vi "Periodic Tasks.vi"(8 "error in (no error)":errorcluster) -> ()   [LabVIEW 2016]
doc: "This VI runs in parallel to other tasks. It can contain as many user-defined periodic loops as you need. These can carry out PID or other sorts of timed response."
uses:
  <vilib>/Rock Robotics/WPI/Utilities/WPI_GetSetVariantRefNum.vi
panel:
  in  "Far Away (2)":u32(colorbox)=16775840
  in  "Far Away":u32(colorbox)=65282
  in  "Lower Value":u32(colorbox)=65282
  in  "Within Limit Distance":u32(colorbox)=65282
  in  "Limit Distance from Sensor":u8(slide)=80 scale=0.0..100.0
  out "sensor":dbl
  out "output variable":dbl
  out "Voltage":dbl
  in  "LED_Off":u32(colorbox)=16775840
  in  "Position Speed":u32(slide)=20 scale=5.0..2000.0
  in  "LED_On":u32(colorbox)=65282
  in  "LED Position":u8(slide)=7 scale=0.0..30.0
  in  "Brightness":u8(slide)=255 scale=0.0..255.0
  out "error out":errorcluster
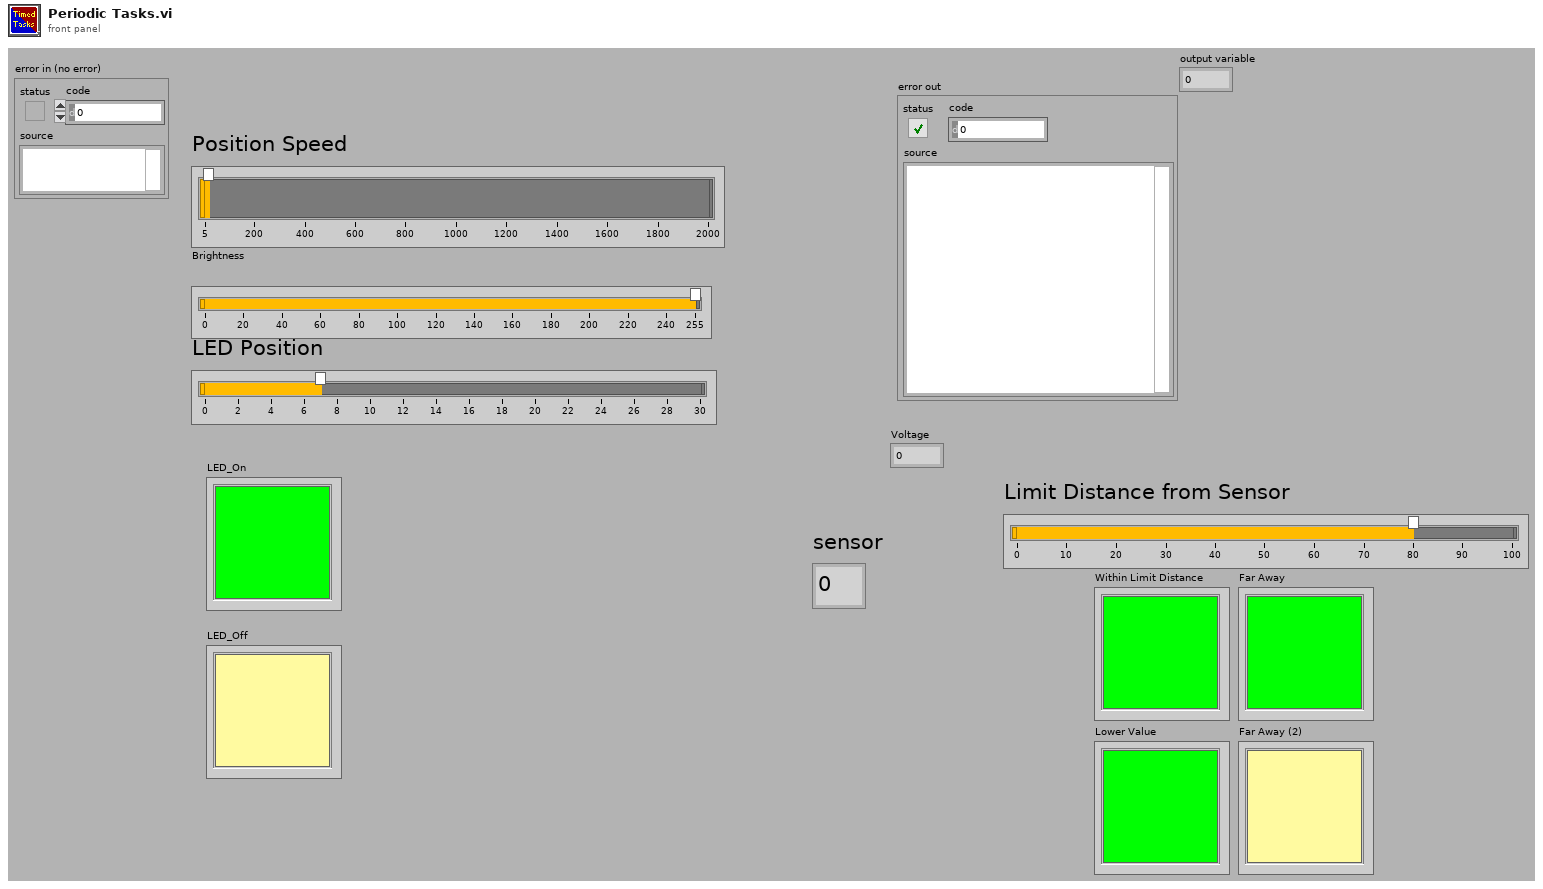
[diagram p1: front panel]
types:
  T1 = typedef "WPI_JoystickDevRef.ctl" = cluster{"Device":T2}
  T2 = typedef "WPI_JoystickDeviceEnum.ctl" = enum16{"USB 0", "USB 1", "USB 2", "USB 3", "USB 4", "USB 5"}
  T3 = typedef "WPI_RobotDriveDevRef.ctl" = cluster{"DevStatus":errorcluster, "Motors[]":T4[], "Square Inputs":bool, "Max Output":dbl}
  T4 = typedef "WPI_MotorControlDeviceRef.ctl" = cluster{"DeviceStatus":errorcluster, "Type":T5, "PWM":cluster{"PWM Channel":T6, "DeadBand":T7}, "CAN":cluster{"Device Number":u8, "SetOutput VI Ref":variant, "GetOutput VI Ref":variant, "Enable VI Ref":variant, "Disable VI Ref":variant, "Data":variant}, "Invert":bool}
  T5 = typedef "WPI_MotorControlType.ctl" = enum16{"PWM", "CAN"}
  T6 = typedef "FPGA_DIOPWMChannel.ctl" = enum8{"PWM 0", "PWM 1", "PWM 2", "PWM 3", "PWM 4", "PWM 5", "PWM 6", "PWM 7", "PWM 8", "PWM 9", "PWM MXP 0", "PWM MXP 1", "PWM MXP 2", "PWM MXP 3", "PWM MXP 4", "PWM MXP 5", "PWM MXP 6", "PWM MXP 7", "PWM MXP 8", "PWM MXP 9", "Invalid"}
  T7 = typedef "WPI_PWMDeadband.ctl" = cluster{"Name":string, "maxPositivePwm":i32, "minPositivePwm":i32, "centerPwm":i32, "maxNegativePwm":i32, "minNegativePwm":i32, "angularRange":u16}
  T8 = typedef "WPI_AnalogChannelDevRef.ctl" = cluster{"DevStatus":errorcluster, "Analog Channel":T9}
  T9 = typedef "FPGA_AIChannel.ctl" = enum8{"AI 0", "AI 1", "AI 2", "AI 3", "AI MXP 0", "AI MXP 1", "AI MXP 2", "AI MXP 3", "Invalid"}
  T10 = cluster{"JoystickDevRef":T1, "RobotDriveDevRef":T3}
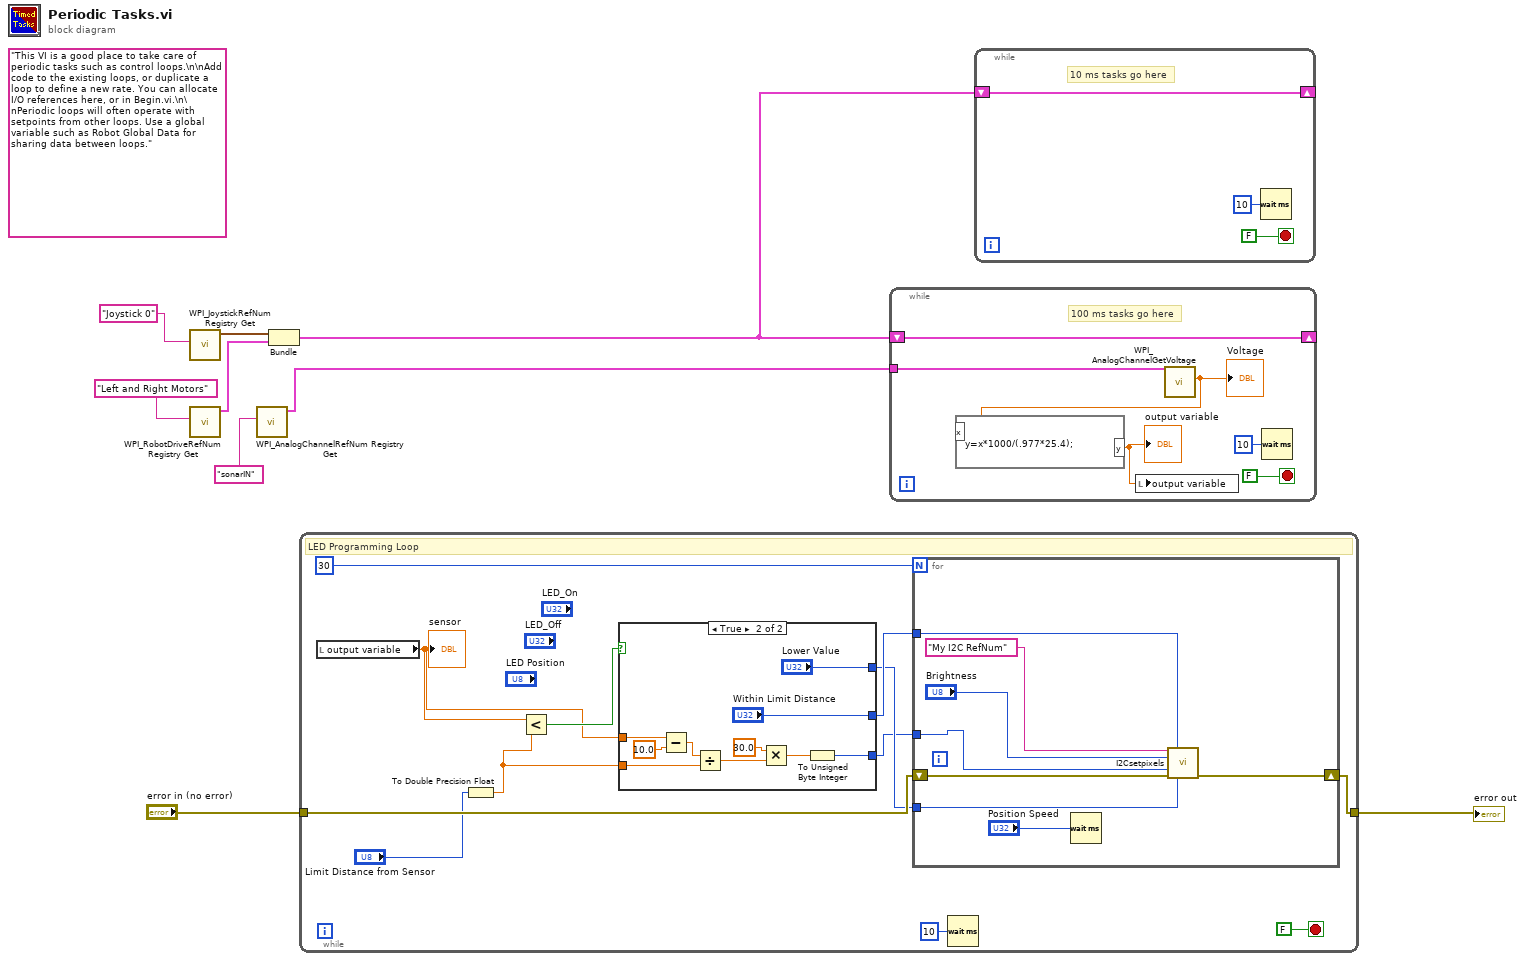
[diagram p0: block diagram]
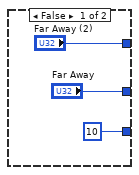
[diagram p2: hidden frame]
diagram:
  (unwired) "This VI is a good place to take care of periodic tasks such as control loops.\n\nAdd code to the existing loops, or duplicate a loop to define a new rate. You can allocate I/O references here, or in Begin.vi.\n\nPeriodic loops will often operate with setpoints from other loops. Use a global variable such as Robot Global Data for sharing data between loops."
  n1 = call <vilib>:"WPI_JoystickRefNum Registry Get.vi"("refnum name"="Joystick 0") -> ("JoystickDevRef"=w7:T1)  [unwired: 1 in, 9 out]
  n2 = call <vilib>:"WPI_RobotDriveRefNum Registry Get.vi"("refnum name"="Left and Right Motors") -> ("RobotDriveDevRef"=w6:T3)  [unwired: 1 in, 9 out]
  n3 = call <vilib>:"WPI_AnalogChannelRefNum Registry Get.vi"("refnum name"="sonarIN") -> ("AIDeviceRef"=w1:T8)  [unwired: 9 in, 1 out]
  n4 = Bundle("JoystickDevRef"=w7, "RobotDriveDevRef"=w6) -> (w5:T10)  [unwired: 1 out]
  n5 = while {
    tunnel: "error in (no error)" -> [w20]
    tunnel: [w17] -> w3
    stop <- FALSE stop-if-true
    # "LED Programming Loop"
    n6 = local read "output variable"() -> (w11:dbl)
    "sensor" <- w11
    n7 = To Double Precision Float(number="Limit Distance from Sensor") -> (double precision float=w10:dbl)
    n8 = Less?(x=w11, y=w10) -> (x < y?=w15:bool)
    n9 = case shown="True" w15 {
      tunnel: ["Far Away" "Within Limit Distance"] -> w14
      tunnel: ["Far Away (2)" "Lower Value"] -> w13
      tunnel: [u8 10 ("LED Position 2") w26] -> w12
      tunnel: w11 -> [_ w32]
      tunnel: w10 -> [_ w29]
      frame False {
      }
      frame True {
        n10 = Subtract(x=w32, y=10.0) -> (x-y=w30:dbl)
        n11 = Divide(x=w30, y=w29) -> (x/y=w28:dbl)
        n12 = Multiply(x=30.0, y=w28) -> (x*y=w25:dbl)
        n13 = To Unsigned Byte Integer(number=w25) -> (unsigned 8bit integer=w26:u8)
      }
    }
    n14 = for {
      N: 30 -> [_]
      shift-right: [w41] -> w17
      shift-left: w20 -> [w42]
      tunnel: w14 -> [w37]
      tunnel: w13 -> [w36]
      tunnel: w12 -> [w35]
      n15 = Wait (ms)(milliseconds to wait="Position Speed") -> ()  [unwired: 1 out]
      n16 = call "I2Csetpixels.vi"("I2C Reference In"="My I2C RefNum" ("refnum name"), "Color Box - On"=w37, "Brightness (0-255)"="Brightness", "LED Position"=w35, "Error In"=w42, "Color Box - Off"=w36) -> ("Error Out"=w41:errorcluster)  [unwired: 8 in, 1 out]
    }
    n17 = Wait (ms)(milliseconds to wait=u32 10) -> ()  [unwired: 1 out]
  }
  "error out" <- w3
  n18 = while {
    shift-right: [w46] -> _
    shift-left: w5 -> [w46]
    tunnel: w1 -> [w45]
    stop <- FALSE stop-if-true
    # "100 ms tasks go here"
    n19 = call <vilib>:"WPI_AnalogChannelGetVoltage.vi"("AIDeviceRef"=w45) -> ("Voltage"=w44:dbl)  [unwired: 8 in, 2 out]
    "Voltage" <- w44
    n20 = formula code="y=x*1000/(.977*25.4);"("x"=w44) -> ("y"=w43:dbl)
    "output variable" <- w43
    n21 = local write "output variable"(w43) -> ()
    n22 = Wait (ms)(milliseconds to wait=u32 10) -> ()  [unwired: 1 out]
  }
  n23 = while {
    shift-right: [w49] -> _
    shift-left: w5 -> [w49]
    stop <- FALSE stop-if-true
    # "10 ms tasks go here"
    n24 = Wait (ms)(milliseconds to wait=u32 10) -> ()  [unwired: 1 out]
  }
